vi "Read.vi"(8 "error in (no error)":errorcluster, 11 "Channel Reader in":refnum<class "Channel Manager.lvclass">) -> (0 "error out":errorcluster, 3 "Channel Reader out":refnum<class "Channel Manager.lvclass">)   [LabVIEW 2024, in "Embedded TDMS Logger Engine.lvlib" / "Channel Manager.lvclass"]
doc: "Read from our channels in VS, check our trigger state and manage that and also set our channel values internally in our File Classes."
uses:
  Channel Manager.lvclass
  Channel Manager.lvclass/Channel Manager.ctl
  <vilib>/NI/NIVS Inline Async API/_Data Access Engine/Access Type Classes/Read/Read.lvclass/Read.ctl
  <vilib>/NI/NIVS Inline Async API/_Data Access Engine/Data Access Engine/Methods/Read.Data.vi
  <vilib>/NI/NIVS Inline Async API/_Data Access Engine/Access Type Classes/Read/Read.ProcessData.vi
  Shared/File Classes/File/File.lvclass
  <vilib>/NI/NIVS Inline Async API/_Data Access Engine/Data Access Engine/Data Access Engine.lvclass
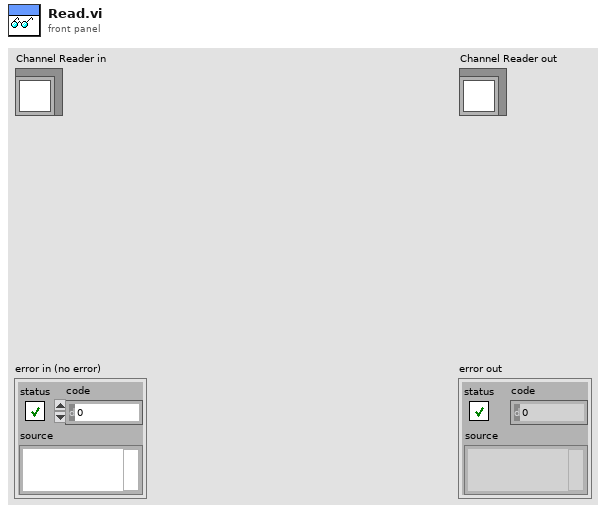
[diagram p1: front panel]
types:
  T1 = typedef "Data Access Engine.lvlib/Data Access Engine.lvclass/Read.DVR.ctl" = refnum<data-value>
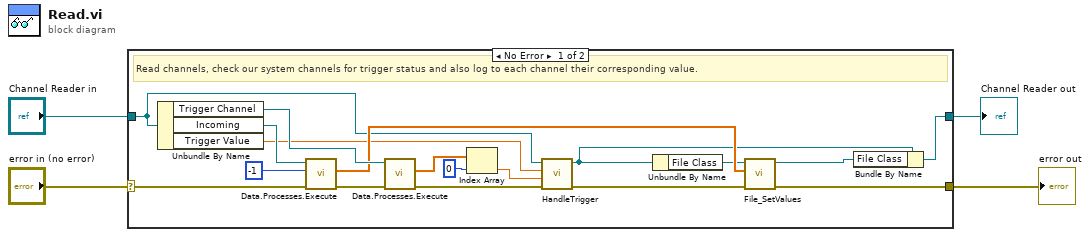
[diagram p0: block diagram]
diagram:
  n1 = case shown="No Error" "error in (no error)" {
    selector: "error in (no error)" -> [w18 w24]
    tunnel: [w16 w24] -> w3
    tunnel: [w15 w23] -> w1
    tunnel: "Channel Reader in" -> [w13 w23]
    frame No Error {
      # "Read channels, check our system channels for trigger status and also log to each channel their corresponding value."
      n2 = Unbundle By Name(w13) -> ("Trigger Channel"=w20:T1, "Incoming"=w19:T1, "Trigger Value"=w7:dbl)
      n3 = call-poly <vilib>:"Data.Processes.Execute.vi"("error in (no error)"=w18, "timeout ms"=-1, "Ref"=w19) -> ("error out"=w22:errorcluster, "Values"=w17:dbl[])  [unwired: 6 in, 1 out]
      n4 = call-poly <vilib>:"Data.Processes.Execute.vi"("error in (no error)"=w22, "Ref"=w20) -> ("error out"=w12:errorcluster, "Values"=w10:dbl[])  [unwired: 7 in, 1 out]
      n5 = Index Array(array=w10, index=0) -> (element=w8:dbl)
      n6 = call-dynamic "HandleTrigger.vi"("error in (no error)"=w12, "Current Trigger Value"=w8, "Previous Trigger Value"=w7, "Channel Manager in"=w13) -> ("error out"=w11:errorcluster, "Channel Manager out"=w5:refnum<class "Channel Manager.lvclass">)  [unwired: 6 in]
      n7 = Unbundle By Name(w5) -> ("File Class"=w6:refnum<class "File.lvclass">)
      n8 = call-dynamic "File_SetValues.vi"("error in (no error)"=w11, "Data In"=w17, "File in"=w6) -> ("error out"=w16:errorcluster, "File out"=w14:refnum<class "File.lvclass">)  [unwired: 7 in]
      n9 = Bundle By Name(cluster=w5, "File Class"=w14) -> (w15:refnum<class "Channel Manager.lvclass">)
    }
    frame Error {
    }
  }
  "error out" <- w3
  "Channel Reader out" <- w1
